vi "Dax_RadValsBP1_2.vi"(11 "Daxsonics":refnum<visa-resource-name>) -> (1 "Freq (MHz)":u16(ring)=1 items=["4", "6", "8", "10", "12", "15", "17", "20", "25", "30", "35", "40", "45", "50"], 2 "Amp (V)":u16(ring) items=["0", "15", "20", "25", "30", "35", "40", "45", "50", "55", "60", "65", "70", "75", "80", "85", "90", "95", "100"], 3 "Gain (dB)":u16(ring) items=["0", "3", "6", "9", "12", "15", "18", "21", "24", "27", "30", "33", "36", "39", "42", "45"])   [LabVIEW 2022 SP3]
uses:
  ScanningControl/Motion Controllers/-MotionRoutines/MotionGlobals.vi
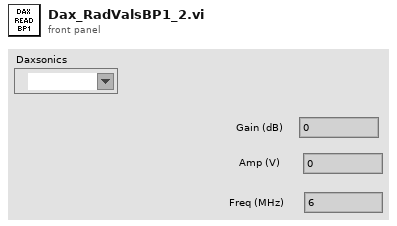
[diagram p1: front panel]
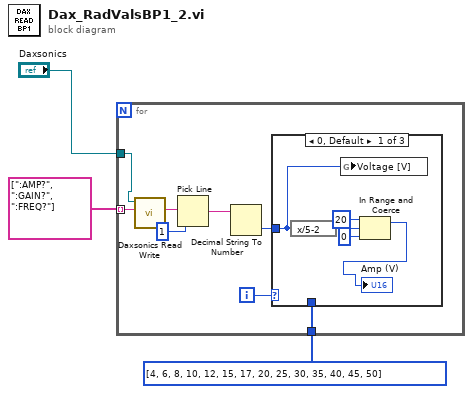
[diagram p0: block diagram]
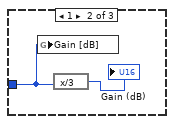
[diagram p2: hidden frame]
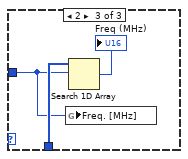
[diagram p3: hidden frame]
diagram:
  n1 = for {
    tunnel: string[] [":AMP?", ":GAIN?", ":FREQ?"] -> [w8] mode=indexing
    tunnel: i32[] [4, 6, 8, 10, 12, 15, 17, 20, 25, 30, 35, 40, 45, 50] -> [w9]
    tunnel: "Daxsonics" -> [w4]
    i -> [w11]
    n2 = call "Daxsonics Read Write.vi"("write buffer"=w8, "VISA resource name"=w4) -> ("read buffer"=w7:string)  [unwired: 7 in, 2 out]
    n3 = Pick Line(multi-line string=w7, line index=1) -> (output string=w6:string)  [unwired: 1 in]
    n4 = Decimal String To Number(string=w6) -> (number=w10:i32)  [unwired: 2 in, 1 out]
    n5 = case shown="0, Default" w11 {
      tunnel: w10 -> [w13 w18 w20]
      tunnel: w9 -> [_ _ w21]
      frame 0, Default {
        n6 = expression code="x/5-2"(w13) -> (w16:i32)
        n7 = global write "MotionGlobals.vi" "Voltage [V]"(w13) -> ()
        n8 = In Range and Coerce(upper limit=20, x=w16, lower limit=0) -> (coerced(x)=→"Amp (V)":i32)  [unwired: 1 out]
      }
      frame 1 {
        n9 = global write "MotionGlobals.vi" "Gain [dB]"(w18) -> ()
        n10 = expression code="x/3"(w18) -> (→"Gain (dB)":i32)
      }
      frame 2 {
        n11 = global write "MotionGlobals.vi" "Freq. [MHz]"(w20) -> ()
        n12 = Search 1D Array(1D array=w21, element=w20) -> (index of element=→"Freq (MHz)":i32)  [unwired: 1 in]
      }
    }
  }
